vi "AdjusteExtremeCurve.vi"(8 "Init Bins Discarded":u32=10, 9 "FFT Size Window":i32=128, 11 "Freq sample":dbl[](array[numeric])) -> (3 "Extended Freq Sample":dbl[](array[numeric]))   [LabVIEW 2014]
uses:
  <vilib>/imath/engines/lvmath2/RunTimeEngine/IndexRead/NIMS V(R2).vi
  <instcachedir>/0/NIMS V(R2)_C76619605A0E4E9F8B2FA9389712AC47.lvgen/NIMS V(R2)_C76619605A0E4E9F8B2FA9389712AC47_000.vi
  <vilib>/imathl/engines/lvmath/Functions/Error Handling/Create Error.vi
  <vilib>/imath/engines/lvmath2/RunTimeEngine/BuiltInFunctions/difference/NIMS_difference(GV,I32).vi
  <instcachedir>/0/NIMS_difference(GV,I32)_DC7351DCBCF840A8AE147F50EC2CE86E.lvgen/NIMS_difference(GV,I32)_DC7351DCBCF840A8AE147F50EC2CE86E_000.vi
  <vilib>/imath/engines/lvmath2/RunTimeEngine/IndexRead/NIMS V(S).vi
  <instcachedir>/0/NIMS V(S)_0488751826AF41519A22953C041130DC.lvgen/NIMS V(S)_0488751826AF41519A22953C041130DC_000.vi
  <vilib>/imath/engines/lvmath2/RunTimeEngine/RangeToken/NIMS_Range.vi
  <instcachedir>/0/NIMS_Range_9BCE657718DF4976A877346C61F22738.lvgen/NIMS_Range_9BCE657718DF4976A877346C61F22738_001.vi
  <vilib>/imath/engines/lvmath2/RunTimeEngine/ErrorHandling/NIMS_Create Error From Enums.vi
  <vilib>/imath/engines/lvmath2/RunTimeEngine/BuiltInFunctions/vconcatmx/NIMS_vconcatmx.vi
  <instcachedir>/0/NIMS_vconcatmx_3F7EE7E265C34A1F815AF13176DC5310.lvgen/NIMS_vconcatmx_3F7EE7E265C34A1F815AF13176DC5310_000.vi
  <vilib>/imath/engines/lvmath2/RunTimeEngine/IndexRead/NIMS M($,S).vi
  <instcachedir>/0/NIMS M($,S)_3E5749BBB62E49528D4765A77F1F6D98.lvgen/NIMS M($,S)_3E5749BBB62E49528D4765A77F1F6D98_000.vi
  <vilib>/imath/engines/lvmath2/RunTimeEngine/NodeEndStatement/NIMS_NodeEndStatement_Output.vi
  <instcachedir>/0/NIMS_NodeEndStatement_Output_53EC0D466D134D7ABD903AC30B43404B.lvgen/NIMS_NodeEndStatement_Output_53EC0D466D134D7ABD903AC30B43404B_005.vi
  <vilib>/imath/engines/lvmath2/RunTimeEngine/ErrorHandling/NIMS_Finalize Error.vi
  <vilib>/imath/engines/lvmath2/RunTimeEngine/BuiltInFunctions/min/1 input/NIMS_min(RV).vi
  <instcachedir>/0/NIMS_min(RV)_EE2DD3E2888846108C5160A664B67832.lvgen/NIMS_min(RV)_EE2DD3E2888846108C5160A664B67832_000.vi
  <vilib>/imath/engines/lvmath2/RunTimeEngine/BuiltInFunctions/abs/NIMS_abs(signed).vi
  <instcachedir>/0/NIMS_abs(signed)_C4FCB8E6058B49B797C7C8D53CA5F6EC.lvgen/NIMS_abs(signed)_C4FCB8E6058B49B797C7C8D53CA5F6EC_000.vi
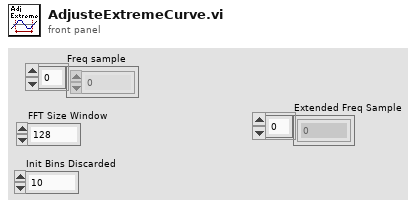
[diagram p1: front panel]
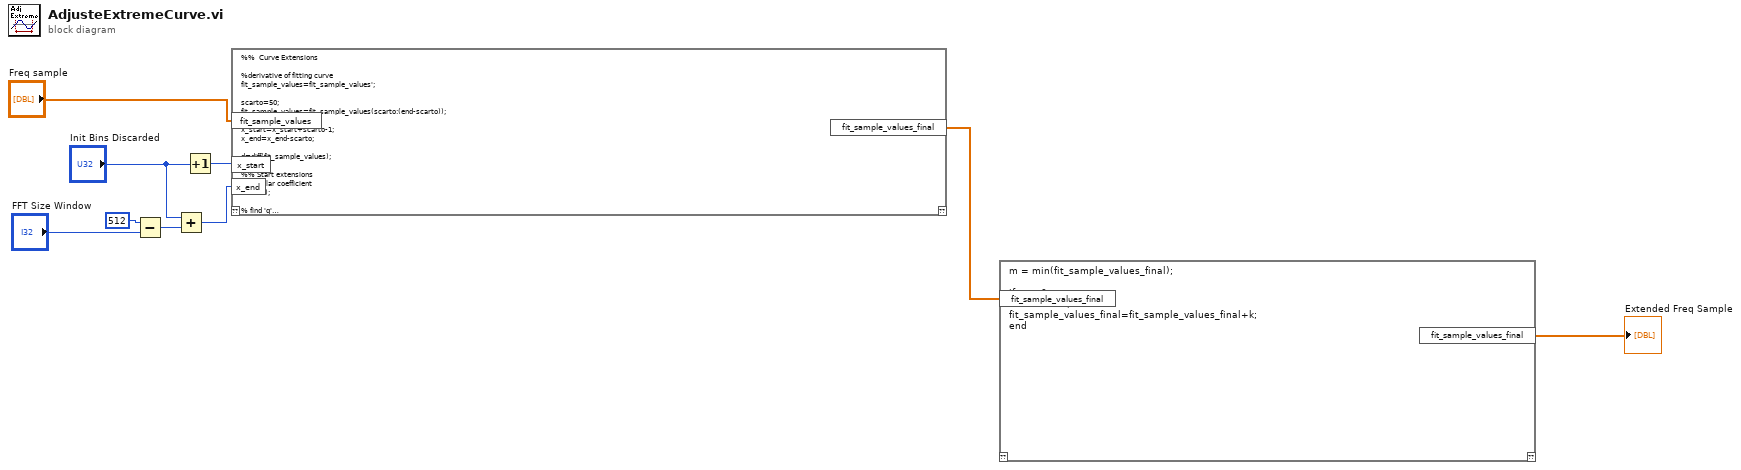
[diagram p0: block diagram]
diagram:
  n1 = Subtract(x=512, y="FFT Size Window") -> (x-y=w6:i32)
  n2 = Add(x="Init Bins Discarded", y=w6) -> (x+y=w5:u32)
  n3 = Increment(x="Init Bins Discarded") -> (x+1=w3:u32)
  n4 = mathscript code="%%  Curve Extensions\n\n%derivative of fitting curve\nfit_sample_values=fit_sample_values';\n\nscarto=50;\nfit_sample_values=fit_sample_values(scarto:(end-scarto));\n\nx_start=x_start+scarto-1;\nx_end=x_end-scarto;\n\nd=diff(fit_sample_values);\n\n%% Start extensions\n% angular coefficient\nm=d(1);\n\n% find 'q'\nx_h=x_start;\nh=fit_sample_values(1);\nq=h-m*x_h;\nx_interval=1:x_start;\n\n% compute line\nretta=m*x_interval+q;\nretta=retta-(retta(end)-fit_sample_values(1));\nfit_sample_values_final=vertcat(retta(1:(end-1))',fit_sample_values);\n\n%% End extension\n% angular coefficient\nm=d(end);\n\n% find 'q'\nx_h=x_end;\nh=fit_sample_values(end);\nq=h-m*x_h;\nx_interval=x_end:625;\n\n% compute line\nretta_2=m*x_interval+q;\nretta_2=retta_2+(fit_sample_values(end)-retta_2(1));\nfit_sample_values_final=vertcat(fit_sample_values_final,retta_2(2:end)');\n\nfit_sample_values_final=fit_sample_values_final(:,1);"("fit_sample_values"="Freq sample", "x_start"=w3, "x_end"=w5) -> ("fit_sample_values_final"=w2:dbl[])  [unwired: 1 in, 1 out]
  n5 = mathscript code="m = min(fit_sample_values_final);\n\nif m < 0\nk=abs(m)*2;\nfit_sample_values_final=fit_sample_values_final+k;\nend"("fit_sample_values_final"=w2) -> ("fit_sample_values_final"=→"Extended Freq Sample":dbl[])  [unwired: 1 in, 1 out]
